vi "Bump Timestamp.vi"(6 "Timestamp (Now)":dbl, 8 "error in (no error)":errorcluster, 11 "Group in":refnum<class "Group DBL.lvclass">) -> (0 "error out":errorcluster, 3 "Group out":refnum<class "Group DBL.lvclass">)   [LabVIEW 2020, in "Vecto.lvlib" / "Group DBL.lvclass"]
uses:
  Group DBL.lvclass
  C:/dev/lv20CE/relink/lv-vecto/Vecto/Group/Group.lvclass
  Group DBL.lvclass/Group DBL.ctl
  Group/Group.lvclass
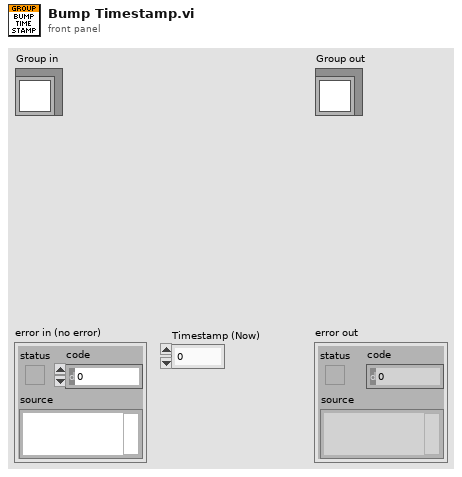
[diagram p1: front panel]
types:
  T1 = typedef "Vecto.lvlib/Group.lvclass/Ref.ctl" = cluster{"Scaled":dbl[], "Timestamp":dbl[], "Raw":dbl[]}
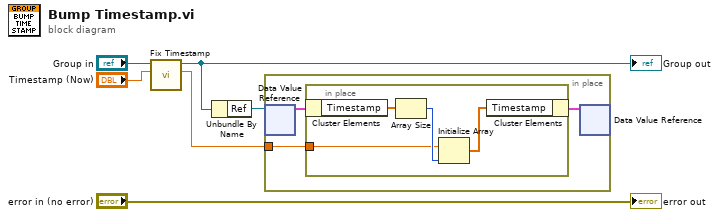
[diagram p0: block diagram]
diagram:
  n1 = call "Fix Timestamp.vi"("Timestamp in"="Timestamp (Now)", "GroupAbstract in"="Group in") -> ("Timestamp"=w1:dbl, "GroupAbstract out"=w2:refnum<class "Group DBL.lvclass">)  [unwired: 7 in, 1 out]
  "Group out" <- w2
  n2 = Unbundle By Name(w2) -> ("Ref"=w3:refnum<data-value>)
  n3 = in-place {
    in-place-border: w1 -> [w7]
    n4 = in-place-dvr #1(w3) -> (w9:T1)  [unwired: 1 out]
    n5 = in-place {
      in-place-border: w7 -> [w10]
      n6 = in-place-cluster #2(w9) -> ("Timestamp"=w13:dbl[])
      n7 = Array Size(array=w13) -> (size(s)=w12:i32)
      n8 = Initialize Array(w10, w12) -> (w11:dbl[])
      n9 = in-place-cluster #2("Timestamp"=w11) -> (w8:T1)
    }
    n10 = in-place-dvr #1(w8) -> ()  [unwired: 2 out]
  }
  "error out" <- "error in (no error)"
